vi "Test T Con.vi"() -> ()   [LabVIEW 2024]
uses:
  NHMFL_Core/Libraries/Instruments/Cryo-con/Cryo-Con Driver/Cryo-Con Driver.lvclass
  Temperature Controller.lvclass
  NHMFL_Core/Libraries/Instruments/Temperature Controller Driver/T controller configuration.ctl
  NHMFL_Core/Libraries/Instruments/Temperature Controller/Controls/Control Mode.ctl
panel:
  in  "Refresh from instrument":bool
  in  "Configuration":T1={"Record Channels"=["A"], "Record raw signal"=FALSE, "Set point"=0.0, "Record heater"=FALSE, "Ramp rate"=0.0, "P"=0.0, "I"=0.0, "D"=0.0, "Control"=enum."Off", "P manual"=0.0, "Output #"=1}
  in  "Stop Button":bool
  out "Temperature":dbl format="%.5f"
  in  "VISA resource name":refnum<visa-resource-name>
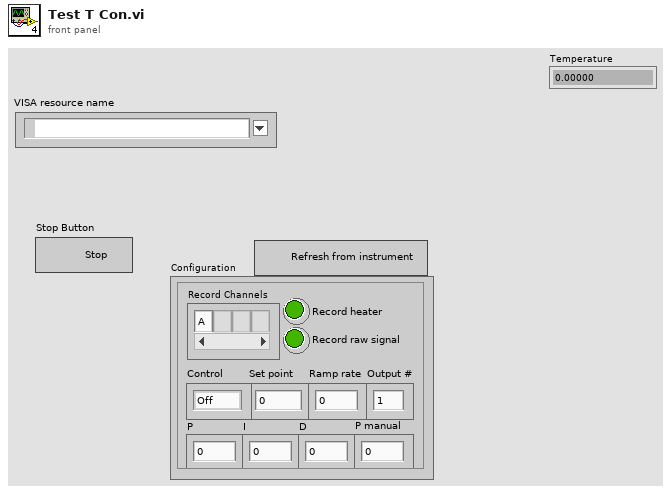
[diagram p1: front panel]
types:
  T1 = typedef "T controller configuration.ctl" = cluster{"Record Channels":string[], "Record raw signal":bool, "Set point":dbl, "Record heater":bool, "Ramp rate":dbl, "P":dbl, "I":dbl, "D":dbl, "Control":T2, "P manual":dbl, "Output #":i32}
  T2 = typedef "Control Mode.ctl" = enum16{"Off", "PID", "Ramp", "Manual", "Table"}
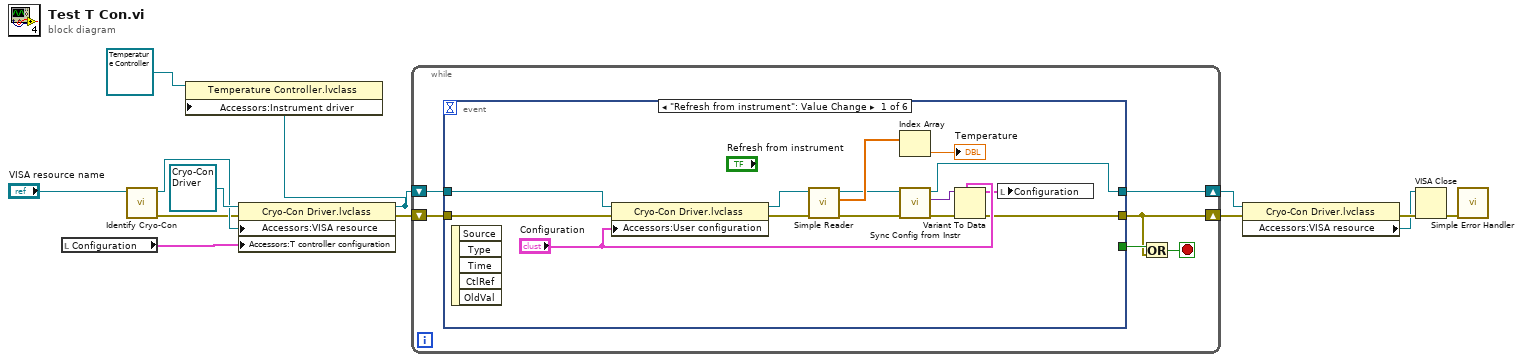
[diagram p0: block diagram]
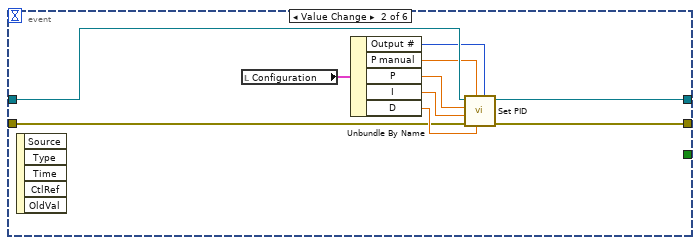
[diagram p2: hidden frame]
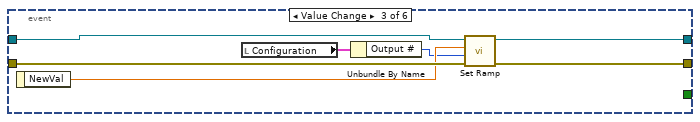
[diagram p3: hidden frame]
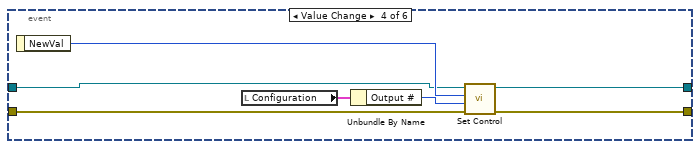
[diagram p4: hidden frame]
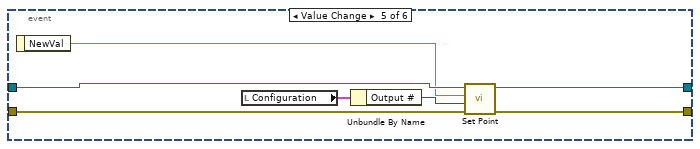
[diagram p5: hidden frame]
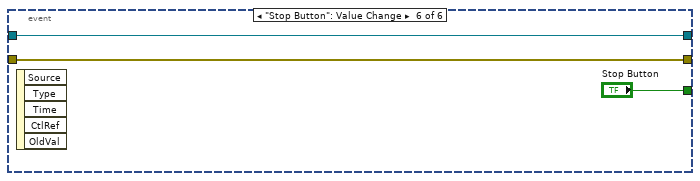
[diagram p6: hidden frame]
diagram:
  n1 = local read "Configuration"() -> (w3:T1)
  n2 = call "Identify Cryo-Con.vi"("VISA resource name"="VISA resource name") -> ("Error Out"=w9:errorcluster, "VISA resource name out"=w10:refnum<visa-resource-name>)  [unwired: 7 in, 2 out]
  n3 = property class="Cryo-Con Driver.lvclass"(reference=refnum<class "Cryo-Con Driver.lvclass"> refnum ("Cryo-Con Driver.lvclass"), error in=w9, "Accessors:VISA resource"=w10, "Accessors:T controller configuration"=w3) -> (reference out=w1:refnum<class "Cryo-Con Driver.lvclass">, error out=w8:errorcluster)
  n4 = property class="Temperature Controller.lvclass"(reference=refnum<class "Temperature Controller.lvclass"> refnum ("Temperature Controller.lvclass"), "Accessors:Instrument driver"=w1) -> ()  [unwired: 1 in, 2 out]
  n5 = while {
    shift-right: [w16] -> w4
    shift-left: w8 -> [w19]
    shift-right: [w14] -> w7
    shift-left: w1 -> [w15]
    stop <- w17 stop-if-true
    n6 = event shown="[0] \"Refresh from instrument\": Value Change" {
      selector: _ -> [_ _ _ _ _ _]
      dyn-events: _ -> [_ _ _ _ _ _]
      timeout: _ -> [_ _ _ _ _ _]
      tunnel: w19 -> [w20 w36 w49 w55 w62 w66]
      tunnel: [w26 w37 w48 w56 w61 w66] -> w16
      tunnel: [_ _ _ _ _ "Stop Button"] -> w18
      tunnel: w15 -> [w24 w43 w50 w53 w64 w65]
      tunnel: [w31 w38 w47 w54 w63 w65] -> w14
      event "Refresh from instrument": Value Change {
        n7 = event-data() -> ()  [unwired: 1 in, 5 out]
        n8 = property class="Cryo-Con Driver.lvclass"(reference=w24, error in=w20, "Accessors:User configuration"="Configuration") -> (reference out=w23:refnum<class "Cryo-Con Driver.lvclass">, error out=w25:errorcluster)
        n9 = call-dynamic "Simple Reader.vi"("error in (no error)"=w25, "Cryo-Con Driver in"=w23) -> ("error out"=w21:errorcluster, "Signals"=w33:dbl[], "Cryo-Con Driver out"=w22:refnum<class "Cryo-Con Driver.lvclass">)  [unwired: 7 in]
        n10 = Index Array(array=w33) -> (element=→"Temperature":dbl)  [unwired: 1 in]
        n11 = call-dynamic "Sync Config from Instr.vi"("error in (no error)"=w21, "Cryo-Con Driver in"=w22) -> ("error out"=w30:errorcluster, "Variant"=w29:variant, "Cryo-Con Driver out"=w31:refnum<class "Cryo-Con Driver.lvclass">)  [unwired: 7 in]
        n12 = Variant To Data(error in=w30, type="Configuration", Variant=w29) -> (data=w27:T1, error out=w26:errorcluster)
        n13 = local write "Configuration"(w27) -> ()
      }
      event Value Change {
        n14 = event-data() -> ()  [unwired: 1 in, 5 out]
        n15 = local read "Configuration"() -> (w42:T1)
        n16 = Unbundle By Name(w42) -> ("Output #"=w34:i32, "P manual"=w35:dbl, "P"=w41:dbl, "I"=w40:dbl, "D"=w39:dbl)
        n17 = call-dynamic "Set PID.vi"("Output #"=w34, "D"=w39, "P manual"=w35, "error in (no error)"=w36, "I"=w40, "P"=w41, "Cryo-Con Driver in"=w43) -> ("error out"=w37:errorcluster, "Cryo-Con Driver out"=w38:refnum<class "Cryo-Con Driver.lvclass">)  [unwired: 3 in]
      }
      event Value Change {
        n18 = event-data() -> ("NewVal"=w46:dbl)  [unwired: 1 in]
        n19 = local read "Configuration"() -> (w45:T1)
        n20 = Unbundle By Name(w45) -> ("Output #"=w44:i32)
        n21 = call-dynamic "Set Ramp.vi"("error in (no error)"=w49, "Output #"=w44, "Ramp rate (0: off)"=w46, "Cryo-Con Driver in"=w50) -> ("error out"=w48:errorcluster, "Cryo-Con Driver out"=w47:refnum<class "Cryo-Con Driver.lvclass">)  [unwired: 6 in]
      }
      event Value Change {
        n22 = event-data() -> ("NewVal"=w57:T2)  [unwired: 1 in]
        n23 = local read "Configuration"() -> (w52:T1)
        n24 = Unbundle By Name(w52) -> ("Output #"=w51:i32)
        n25 = call-dynamic "Set Control.vi"("error in (no error)"=w55, "Output #"=w51, "Control"=w57, "Cryo-Con Driver in"=w53) -> ("error out"=w56:errorcluster, "Cryo-Con Driver out"=w54:refnum<class "Cryo-Con Driver.lvclass">)  [unwired: 6 in]
      }
      event Value Change {
        n26 = event-data() -> ("NewVal"=w60:dbl)  [unwired: 1 in]
        n27 = local read "Configuration"() -> (w59:T1)
        n28 = Unbundle By Name(w59) -> ("Output #"=w58:i32)
        n29 = call-dynamic "Set Point.vi"("error in (no error)"=w62, "Output #"=w58, "Set point"=w60, "Cryo-Con Driver in"=w64) -> ("error out"=w61:errorcluster, "Cryo-Con Driver out"=w63:refnum<class "Cryo-Con Driver.lvclass">)  [unwired: 6 in]
      }
      event "Stop Button": Value Change {
        n30 = event-data() -> ()  [unwired: 1 in, 5 out]
      }
    }
    n31 = Or(x=w18, y=w16) -> (x .or. y?=w17:bool)
  }
  n32 = property class="Cryo-Con Driver.lvclass"(reference=w7, error in=w4) -> (error out=w6:errorcluster, "Accessors:VISA resource"=w5:refnum<visa-resource-name>)  [unwired: 1 out]
  n33 = VISA Close(VISA resource name=w5, error in (no error)=w6) -> (error out=w13:errorcluster)
  n34 = call <vilib>:"Simple Error Handler.vi"("error in (no error)"=w13) -> ()  [unwired: 4 in, 5 out]
